vi "Generar.vi"(8 "error in (no error)":errorcluster, 11 "Generador in":refnum<class "Generador.lvclass">) -> (0 "error out":errorcluster)   [LabVIEW 2020, in "Generador.lvlib" / "Generador.lvclass"]
uses:
  Generador.lvclass
  Generador.lvclass/Generador.ctl
  Log/Log Messages/Save to file Msg/Save to file Msg.lvclass/Save to file Msg.ctl
  <vilib>/ActorFramework/Message Enqueuer/Message Enqueuer.lvclass/Message Enqueuer.ctl
  <vilib>/ActorFramework/Message Enqueuer/Enqueue.vi
  Log/Log Messages/Save to file Msg/Save to file Msg.lvclass
  C:/Program Files (x86)/National Instruments/LabVIEW 2020/vi.lib/ActorFramework/Message/Message.lvclass
  <vilib>/ActorFramework/Message Priority Queue/Priority Enqueue.vi
  <vilib>/measure/NI_MABase.lvlib
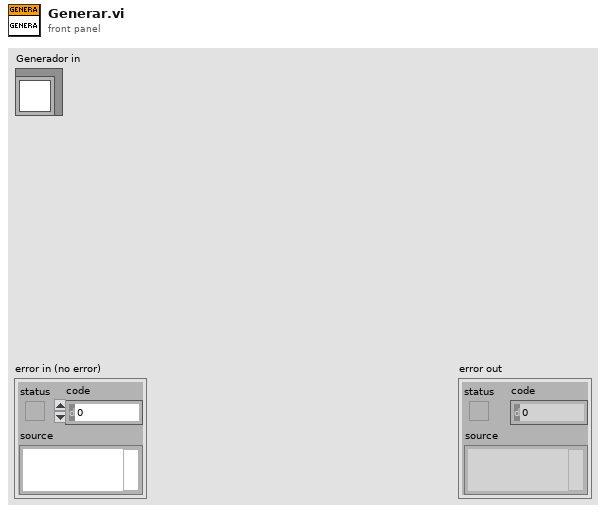
[diagram p1: front panel]
types:
  T1 = cluster{"offset":dbl, "square wave duty cycle (%)":dbl, "reset signal":bool, "sampling info":cluster{"Fs":dbl, "#s":dbl}, "phase":dbl, "signal type":enum16{"Sine Wave", "Triangle Wave", "Square Wave", "Sawtooth Wave"}, "amplitude":dbl, "frequency":dbl}
  T2 = enum16{"Sine Wave", "Triangle Wave", "Square Wave", "Sawtooth Wave"}
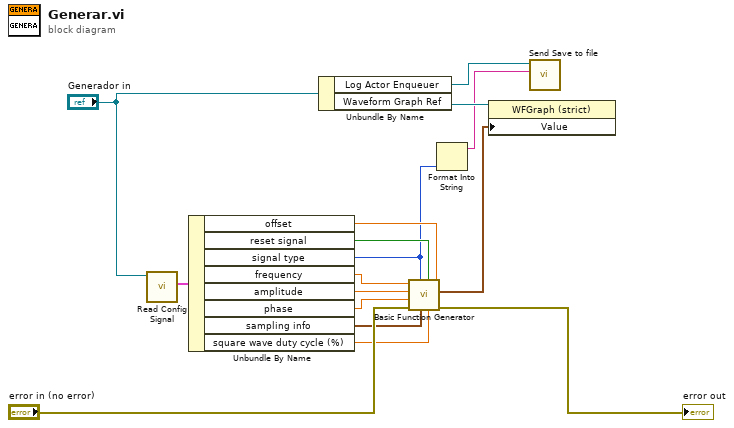
[diagram p0: block diagram]
diagram:
  n1 = call "Read Config Signal.vi"("Generador in"="Generador in") -> ("Config Signal"=w14:T1)  [unwired: 8 in, 2 out]
  n2 = Unbundle By Name(w14) -> ("offset"=w13:dbl, "reset signal"=w12:bool, "signal type"=w3:T2, "frequency"=w11:dbl, "amplitude"=w10:dbl, "phase"=w9:dbl, "sampling info"=w8:cluster{"Fs":dbl, "#s":dbl}, "square wave duty cycle (%)"=w7:dbl)
  n3 = Unbundle By Name("Generador in") -> ("Log Actor Enqueuer"=w4:refnum<class "Message Enqueuer.lvclass">, "Waveform Graph Ref"=w5:refnum<vi>)
  n4 = call <vilib>:"Basic Function Generator.vi"("offset"=w13, "square wave duty cycle (%)"=w7, "reset signal"=w12, "sampling info"=w8, "signal type"=w3, "error in (no error)"="error in (no error)", "phase"=w9, "amplitude"=w10, "frequency"=w11) -> ("error out"=→"error out":errorcluster, "signal out"=w1:waveform(dbl))  [unwired: 1 out]
  n5 = Format Into String(w3) -> (resulting string=w2:string)  [unwired: 3 in, 1 out]
  n6 = property class="WFGraph (strict)"(reference=w5, "Value"=w1) -> ()  [unwired: 1 in, 2 out]
  n7 = call "Send Save to file.vi"("Sent By"=w2, "Message Enqueuer"=w4) -> ()  [unwired: 8 in, 2 out]
